vi "uvod.vi"() -> ()   [LabVIEW 2025]
panel:
  in  "stop":bool
  out "Waveform Graph":waveform(dbl)(graph)
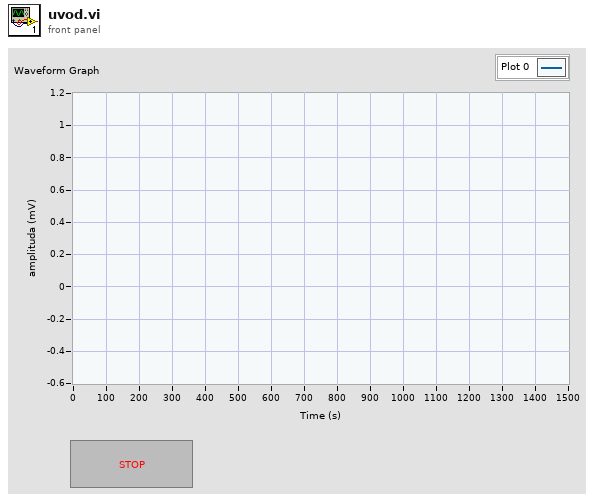
[diagram p1: front panel]
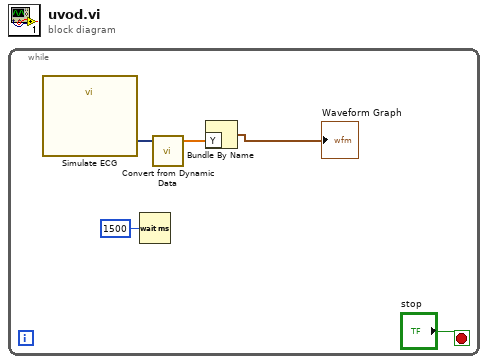
[diagram p0: block diagram]
diagram:
  n1 = while {
    stop <- "stop" stop-if-true
    n2 = call "Simulate ECG"() -> ("ECG"=w3:dynamicdata)  [unwired: 10 in, 1 out]
    n3 = Wait (ms)(milliseconds to wait=u32 1500) -> ()  [unwired: 1 out]
    n4 = call "Convert from Dynamic Data"("Dynamic Data Type"=w3) -> ("Array"=w4:dbl[])  [unwired: 3 in]
    n5 = Bundle By Name("Y"=w4) -> (→"Waveform Graph":waveform(dbl))  [unwired: 1 in]
  }
